vi "DB - [MasterData].[OutputSet].vi"(5 "Master Data OuputSet SQL":T1, 7 "DB Connection":T3={"Open"=TRUE, "Close"=TRUE}, 8 "error in (no error)":errorcluster, 9 "[PlantId]":string, 10 "[OutputSetId]":string, 11 "connection reference":T2) -> (0 "SUMMARY":errorcluster, 1 "Template Files":string[](array[string]), 2 "2D data":string[][](array[string]), 3 "connection reference":T2, 4 "[LayoutId]":string[](array[string]))   [LabVIEW 2013]
uses:
  <vilib>/addons/database/Connection.llb/Conn ObjectReference.ctl
  Controls/DB - OpenClose.ctl
  Controls/DB - Master Data OutputSet SQL.ctl
  Controls/Global SRTRS.vi
  <vilib>/addons/database/Connection.llb/DB Tools Open Connec (String).vi
  <vilib>/addons/database/NI_Database_API.lvlib
panel:
  in  "SRTRS.MasterData.Layout":string="SRTRS.MasterData.Layout"
  in  "SRTRS.MasterData.OutputLayout":string="SRTRS.MasterData.OutputLayout"
  out "Close":errorcluster
  out "SQL Statement":string
  in  "SRTRS.MasterData.OutputSet":string="SRTRS.MasterData.OutputSet"
  out "Connection Information":T4={"Connection "="SQL Server 32bit HPEnvy", "Username"="admin", "Password"="admin123"}
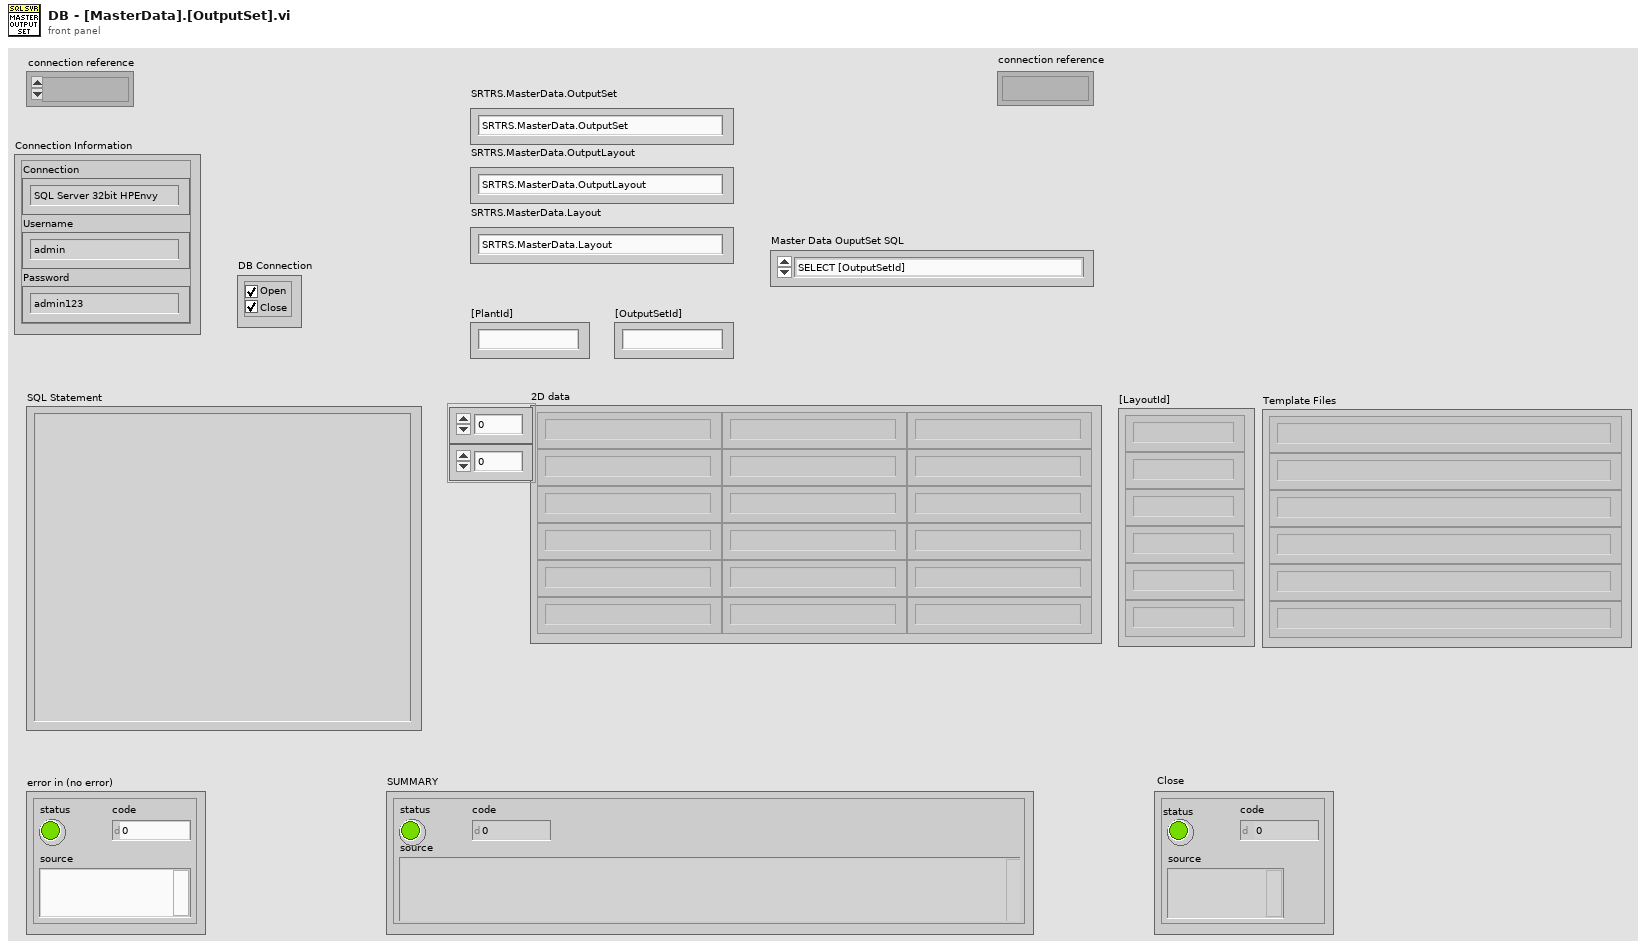
[diagram p1: front panel]
types:
  T1 = typedef "DB - Master Data OutputSet SQL.ctl" = enum16{"SELECT [OutputSetId]", "SELECT [LayoutFilePath],[LayoutFileName]"}
  T2 = typedef "NI_Database_API.lvlib/Conn ObjectReference.ctl" = refnum<k1>
  T3 = typedef "DB - OpenClose.ctl" = cluster{"Open":bool, "Close":bool}
  T4 = cluster{"Connection ":string, "Username":string, "Password":string}
  T5 = typedef "Enum - InteractiveMode-SubVIMode.ctl" = enum16{"Interactive", "subVI Mode"}
  T6 = typedef "Connection Information Cluster.ctl" = cluster{"Connection ":string, "Username":string, "Password":string}
  T7 = typedef "DB - DB.Schema.Table.ctl" = cluster{"DB":string, "Schema":string, "Table":string}
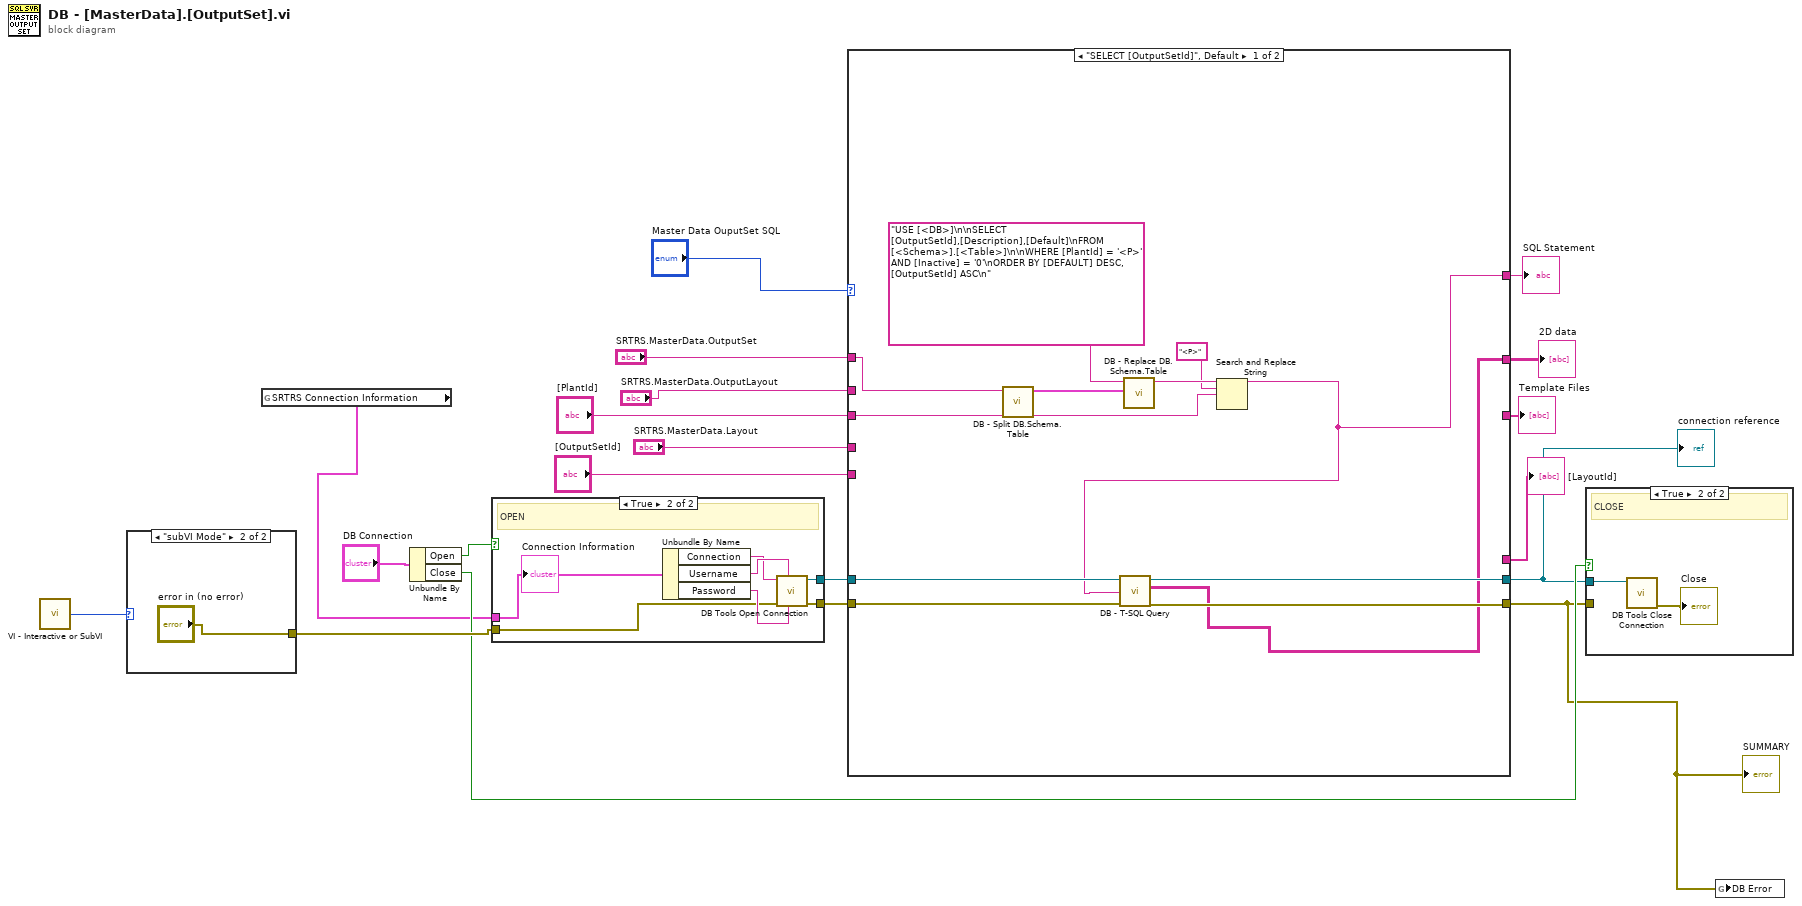
[diagram p0: block diagram]
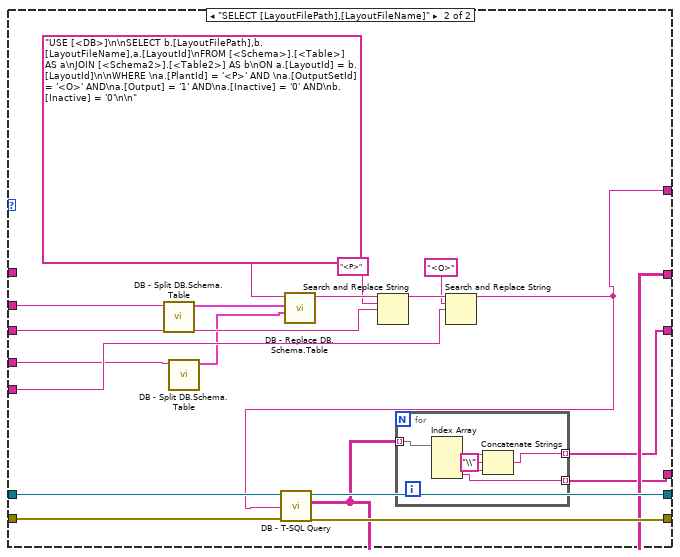
[diagram p2: hidden frame]
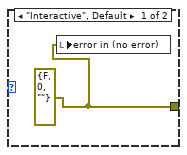
[diagram p4: hidden frame]
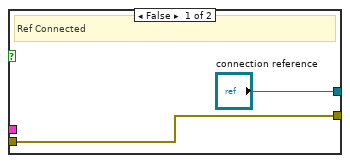
[diagram p5: hidden frame]
diagram:
  n1 = call "VI - Interactive or SubVI.vi"() -> ("Mode"=w18:T5)  [unwired: 5 in]
  n2 = case shown="\"subVI Mode\"" w18 {
    tunnel: [w21 "error in (no error)"] -> w17
    frame "Interactive", Default {
      w21 = errorcluster {"status"=FALSE, "code"=0, "source"=""} ("error in (no error)")
      n3 = local write "error in (no error)"(w21) -> ()
    }
    frame "subVI Mode" {
    }
  }
  n4 = global read "Global SRTRS.vi" "SRTRS Connection Information"() -> (w13:T6)
  n5 = Unbundle By Name("DB Connection") -> ("Open"=w19:bool, "Close"=w16:bool)
  n6 = case shown="True" w19 {
    tunnel: ["connection reference" w28] -> w12
    tunnel: w17 -> [w23 w27]
    tunnel: [w23 w26] -> w11
    tunnel: w13 -> [_ w25]
    frame False {
      # "Ref Connected"
    }
    frame True {
      # "OPEN"
      n7 = Unbundle By Name(w25) -> ("Connection"=w30:string, "Username"=w31:string, "Password"=w29:string)
      n8 = call-poly <vilib>:"DB Tools Open Connection.vi"("password"=w29, "userID"=w31, "error in (no error)"=w27, "connection information"=w30) -> ("error out"=w26:errorcluster, "connection reference"=w28:T2)  [unwired: 4 in]
      "Connection Information" <- w25
    }
  }
  n9 = case shown="\"SELECT [OutputSetId]\", Default" "Master Data OuputSet SQL" {
    tunnel: "[PlantId]" -> [w40 w59]
    tunnel: "SRTRS.MasterData.OutputSet" -> [w39 _]
    tunnel: w12 -> [w37 w57]
    tunnel: w11 -> [w36 w56]
    tunnel: [w35 w55] -> w10
    tunnel: [w34 w54] -> w9
    tunnel: [w33 w48] -> w8
    tunnel: [w32 w52] -> w6
    tunnel: "[OutputSetId]" -> [_ w50]
    tunnel: "SRTRS.MasterData.OutputLayout" -> [_ w49]
    tunnel: [_ w47] -> w3
    tunnel: "SRTRS.MasterData.Layout" -> [_ w46]
    tunnel: [_ w44] -> w1
    frame "SELECT [OutputSetId]", Default {
      n10 = call "DB - Split DB.Schema.Table.vi"("DB.Schema.Table"=w39) -> ("DB.Schema.Table"=w43:T7)  [unwired: 10 in]
      n11 = call "DB - Replace DB.Schema.Table.vi"("DB.Schema.Table"=w43, "string in"="USE [<DB>]\n\nSELECT [OutputSetId],[Description],[Default]\nFROM [<Schema>].[<Table>]\n\nWHERE [PlantId] = '<P>' AND [Inactive] = '0'\nORDER BY [DEFAULT] DESC, [OutputSetId] ASC\n") -> ("string out"=w42:string)  [unwired: 8 in, 1 out]
      n12 = Search and Replace String(input string=w42, search string="<P>", replace string=w40) -> (result string=w32:string)  [unwired: 5 in, 3 out]
      n13 = call "DB - T-SQL Query.vi"("error in (no error)"=w36, "T-SQL"=w32, "connection reference"=w37) -> ("error out"=w34:errorcluster, "2D data"=w33:string[][], "connection reference"=w35:T2)  [unwired: 6 in]
    }
    frame "SELECT [LayoutFilePath],[LayoutFileName]" {
      n14 = call "DB - Split DB.Schema.Table.vi"("DB.Schema.Table"=w49) -> ("DB.Schema.Table"=w62:T7)  [unwired: 10 in]
      n15 = call "DB - Split DB.Schema.Table.vi"("DB.Schema.Table"=w46) -> ("DB.Schema.Table"=w45:T7)  [unwired: 10 in]
      n16 = call "DB - Replace DB.Schema.Table.vi"("DB.Schema.Table 2"=w45, "DB.Schema.Table"=w62, "string in"="USE [<DB>]\n\nSELECT b.[LayoutFilePath],b.[LayoutFileName],a.[LayoutId]\nFROM [<Schema>].[<Table>] AS a\nJOIN [<Schema2>].[<Table2>] AS b\nON a.[LayoutId] = b.[LayoutId]\n\nWHERE \na.[PlantId] = '<P>' AND \na.[OutputSetId] = '<O>' AND\na.[Output] = '1' AND\na.[Inactive] = '0' AND\nb.[Inactive] = '0'\n\n") -> ("string out"=w61:string)  [unwired: 7 in, 1 out]
      n17 = Search and Replace String(input string=w61, search string="<P>", replace string=w59) -> (result string=w53:string)  [unwired: 5 in, 3 out]
      n18 = Search and Replace String(input string=w53, search string="<O>", replace string=w50) -> (result string=w52:string)  [unwired: 5 in, 3 out]
      n19 = call "DB - T-SQL Query.vi"("error in (no error)"=w56, "T-SQL"=w52, "connection reference"=w57) -> ("error out"=w54:errorcluster, "2D data"=w48:string[][], "connection reference"=w55:T2)  [unwired: 6 in]
      n20 = for {
        tunnel: w48 -> [w68] mode=indexing
        tunnel: [w65] -> w47 mode=indexing
        tunnel: [w63] -> w44 mode=indexing
        n21 = Index Array(array=w68) -> (element #1=w67:string, element #2=w66:string, element #3=w63:string)  [unwired: 3 in]
        n22 = Concatenate Strings(w67, "\\" ("string"), w66) -> (w65:string)
      }
    }
  }
  "SUMMARY" <- w9
  "connection reference" <- w10
  "2D data" <- w8
  "SQL Statement" <- w6
  "Template Files" <- w3
  "[LayoutId]" <- w1
  n23 = case shown="True" w16 {
    tunnel: w10 -> [_ w70]
    tunnel: w9 -> [_ _]
    frame False {
      # "Ref Connected"
    }
    frame True {
      # "CLOSE"
      n24 = call <vilib>:"DB Tools Close Connection.vi"("connection reference"=w70) -> ("error out"=→"Close":errorcluster)  [unwired: 6 in]
    }
  }
  n25 = global write "Global SRTRS.vi" "DB Error"(w9) -> ()
